vi "Write VI Plain Name.vi"(8 "error in (no error)":errorcluster, 10 "VI Plain Name":string, 11 "VI in":refnum<class "VI.lvclass">) -> (0 "error out":errorcluster, 3 "VI out":refnum<class "VI.lvclass">)   [LabVIEW 2019, in "VI.lvclass"]
uses:
  VI.lvclass
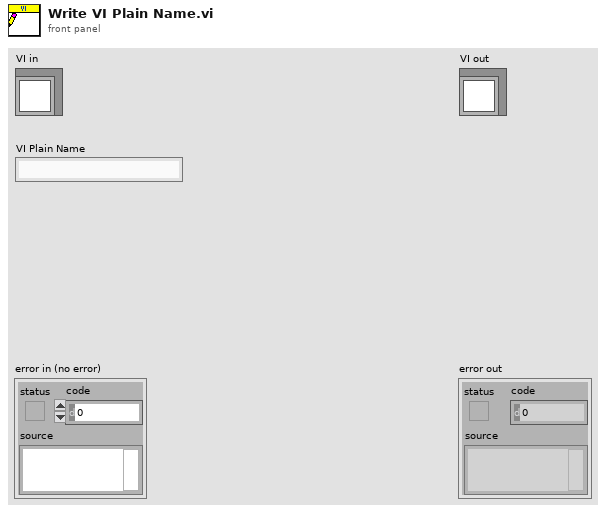
[diagram p1: front panel]
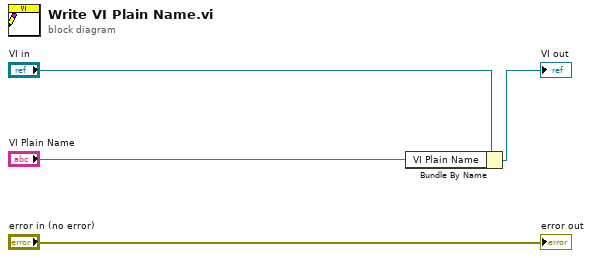
[diagram p0: block diagram]
diagram:
  n1 = Bundle By Name(cluster="VI in", "VI Plain Name"="VI Plain Name") -> (→"VI out":refnum<class "VI.lvclass">)
  "error out" <- "error in (no error)"
